vi "chat completions (OpenAI).vi"(6 "timeout (600000)":i32=600000, 8 "error in":errorcluster, 9 "chat-completion req":T2={"model"="", "messages"=[], "max_tokens"=0, "temperature"=0.0, "stream"=FALSE, "reasoning"={"effort"=enum."low", "exclude"=FALSE}}, 10 "API url":string, 11 "Refnum in":T3) -> (0 "error out":errorcluster, 1 "previous messages":T1[](array[typedef]), 2 "Answer content":string, 3 "Refnum out":T3, 4 "reasoning content":string)   [LabVIEW 2023, in "LabVIEW LLM.lvlib"]
uses:
  LabVIEW LLM.lvlib
  <vilib>/httpClient/ClientHandle.ctl
  chat-completion req.ctl
  openai_message.ctl
  <vilib>/httpClient/POSTBuffer.vi
  <vilib>/httpClient/LabVIEWHTTPClient.lvlib
  <vilib>/addons/_JKI.lib/Serialization/JSON/JKI JSON Serialization.lvlib
  labview-ai-share/LabVIEW AI Base.lvlib
panel:
  out "Request JSON":string
  out "Response JSON":string
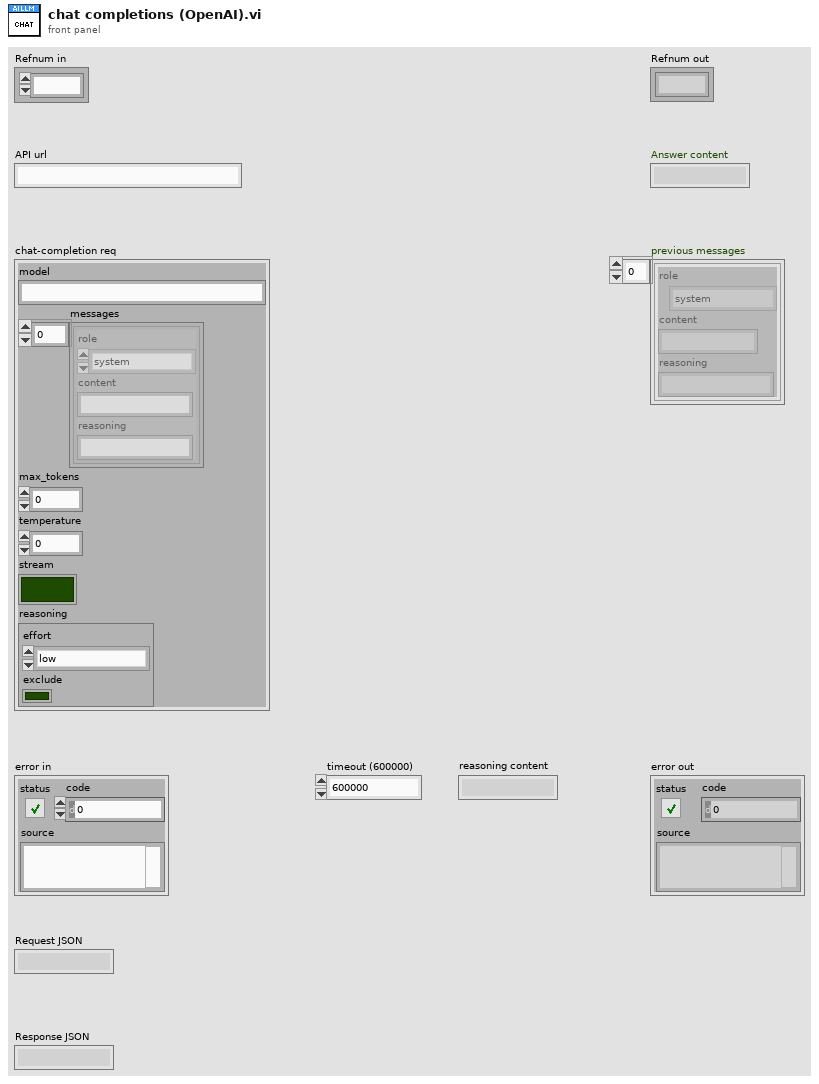
[diagram p1: front panel]
types:
  T1 = typedef "LabVIEW LLM.lvlib/openai_message.ctl" = cluster{"role":enum16{"system", "user", "assistant"}, "content":string, "reasoning":string}
  T2 = typedef "LabVIEW LLM.lvlib/chat-completion req.ctl" = cluster{"model":string, "messages":T1[], "max_tokens":u32, "temperature":dbl, "stream":bool, "reasoning":cluster{"effort":enum16{"high", "medium", "low"}, "exclude":bool}}
  T3 = typedef "LabVIEWHTTPClient.lvlib/ClientHandle.ctl" = refnum<k1>
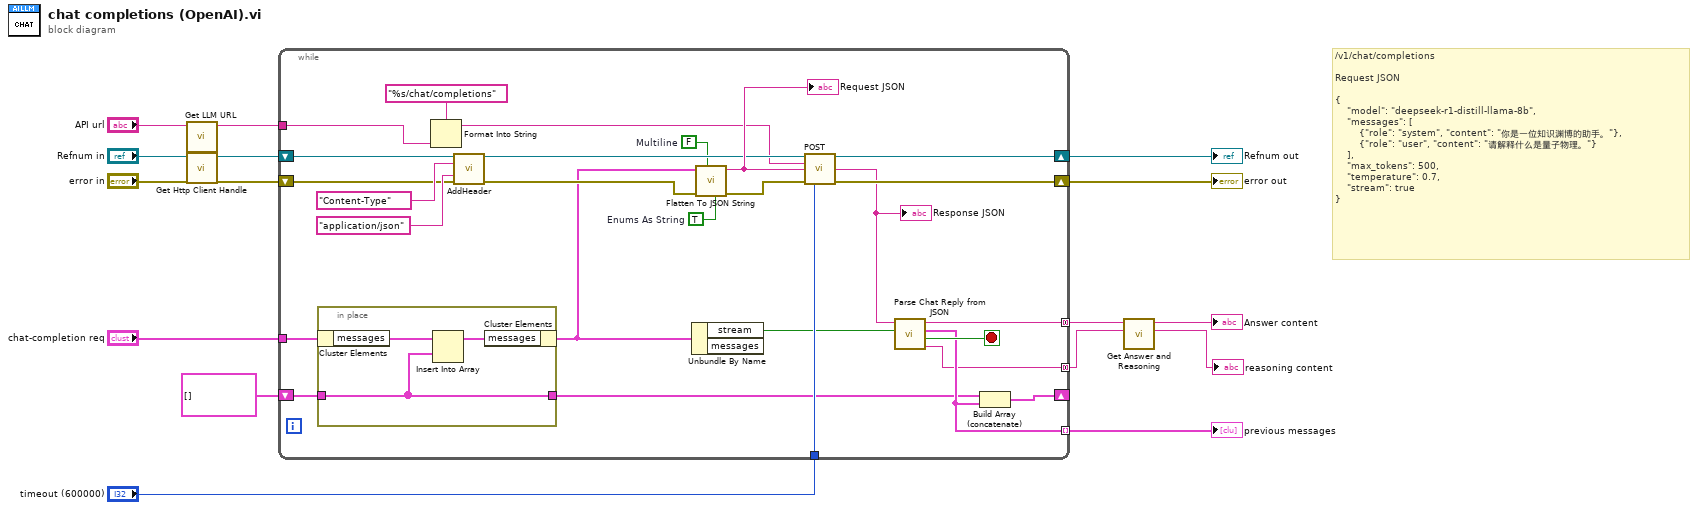
[diagram p0: block diagram]
diagram:
  # "/v1/chat/completions\n\nRequest JSON\n\n{\n    \"model\": \"deepseek-r1-distill-llama-8b\",\n    \"messages\": [\n        {\"role\": \"system\", \"content\": \"你是一位知识渊博的助手。\"},\n        {\"role\": \"user\", \"content\": \"请解释什么是量子物理。\"}\n    ],\n    \"max_tokens\": 500,\n    \"temperature\": 0.7,\n    \"stream\": true\n}"
  n1 = call "Get LLM URL.vi"("OpenAI API URL"="API url") -> ("OpenAI API URL"=w5:string)  [unwired: 10 in]
  n2 = call "Get Http Client Handle.vi"("Refnum in"="Refnum in") -> ("Refnum out"=w4:T3)  [unwired: 10 in]
  n3 = while {
    tunnel: "timeout (600000)" -> [w42]
    tunnel: "chat-completion req" -> [w33]
    tunnel: w5 -> [w30]
    shift-right: [w34] -> w12
    shift-left: w4 -> [w36]
    shift-right: [w41] -> w14
    shift-left: "error in" -> [w31]
    tunnel: [w23] -> w8 mode=concatenating
    shift-right: [w18] -> _
    shift-left: T1[] [] ("Array") -> [w22]
    tunnel: [w21] -> w6 mode=indexing
    tunnel: [w16] -> w3 mode=concatenating
    stop <- w24 stop-if-true
    w26 = TRUE  # Enums As String
    w27 = FALSE  # Multiline
    n4 = in-place {
      in-place-border: w22 -> [w43]
      in-place-border: [w43] -> w17
      n5 = in-place-cluster #1(w33) -> ("messages"=w45:T1[])
      n6 = Insert Into Array(array=w45, new element=w43) -> (w44:T1[])  [unwired: 1 in]
      n7 = in-place-cluster #1("messages"=w44) -> (w20:T2)
    }
    n8 = Format Into String(format string="%s/chat/completions" ("url"), w30) -> (resulting string=w28:string)  [unwired: 2 in, 1 out]
    n9 = call <vilib>:"AddHeader.vi"("client handle"=w36, "header"="Content-Type", "value"="application/json", "error in (no error)"=w31) -> ("client handle out"=w37:T3, "error out"=w35:errorcluster)  [unwired: 10 in]
    n10 = Unbundle By Name(w20) -> ("stream"=w19:bool)  [unwired: 1 out]
    n11 = call <vilib>:"Flatten To JSON String.vi"("Enums As String (F)"=w26, "Multiline (T)"=w27, "error in (no error)"=w35, "Variant"=w20) -> ("error out"=w32:errorcluster, "JSON String"=w40:string)  [unwired: 6 in]
    "Request JSON" <- w40
    n12 = call-poly <vilib>:"POST.vi"("client handle"=w37, "url"=w28, "buffer"=w40, "error in (no error)"=w32, "timeout (10000)"=w42) -> ("client handle out"=w34:T3, "body"=w25:string, "error out"=w41:errorcluster)  [unwired: 7 in, 1 out]
    "Response JSON" <- w25
    n13 = call "Parse Chat Reply from JSON.vi"("stream"=w19, "Response JSON"=w25) -> ("openrouter reasoning"=w16:string, "complete?"=w24:bool, "message"=w21:T1, "answer"=w23:string)  [unwired: 6 in]
    n14 = Build Array (concatenate)(w17, w21) -> (w18:T1[])
  }
  "error out" <- w14
  "Refnum out" <- w12
  "previous messages" <- w6
  n15 = call "Get Answer and Reasoning.vi"("openrouter reasoning"=w3, "answer"=w8) -> ("reasoning"=→"reasoning content":string, "answer"=→"Answer content":string)  [unwired: 8 in]
